vi "Example Code.vi"   [LabVIEW 2016]
uses:
  <vilib>/Skyline/Configuration/Configuration HTTP_class/Open Configuration HTTP.vi
  <vilib>/Skyline/Message/HTTP Wrapper/Open (HTTP).vi
  <vilib>/Skyline/Message/HTTP Wrapper/NI Skyline Message HTTP.lvclass
  <vilib>/Skyline/Configuration/Configuration HTTP_class/NI Skyline Configuration HTTP.lvclass
  <vilib>/Skyline/Message/NI Skyline Message.lvclass
  <vilib>/Skyline/Configuration/Configuration_class/NI Skyline Configuration.lvclass
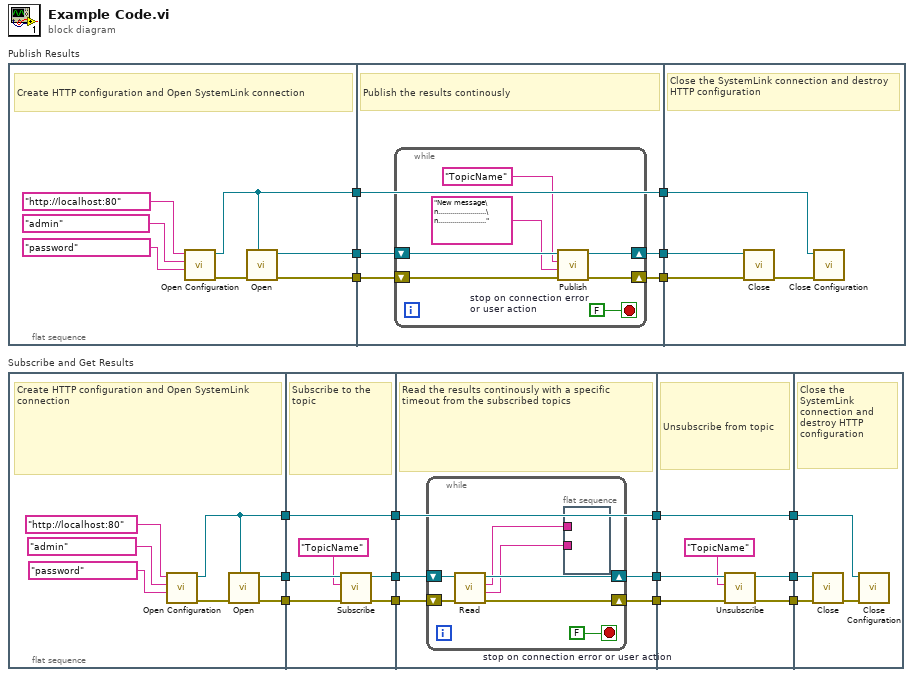
[diagram p0: block diagram]
diagram:
  n1 = flat-sequence "Publish Results" {
    tunnel: [w21] -> w18
    tunnel: [w20] -> w17
    tunnel: [w19] -> w16
    tunnel: w18 -> [w30]
    tunnel: w17 -> [w29]
    tunnel: w16 -> [w28]
    tunnel: [w28] -> w15
    tunnel: [w27] -> w14
    tunnel: [w26] -> w13
    tunnel: w15 -> [w38]
    tunnel: w14 -> [w39]
    tunnel: w13 -> [w40]
    frame #0 {
      # "Create HTTP configuration and Open SystemLink connection"
      n2 = call-poly <vilib>:"Open Configuration.vi"("password"="password", "username"="admin", "server url"="http://localhost:80") -> ("error out"=w25:errorcluster, "HTTP configuration out"=w19:refnum<class "NI Skyline Configuration HTTP.lvclass">)  [unwired: 7 in]
      n3 = call-poly <vilib>:"Open.vi"("configuration"=w19, "error in (no error)"=w25) -> ("error out"=w20:errorcluster, "message http out"=w21:refnum<class "NI Skyline Message HTTP.lvclass">)  [unwired: 8 in]
    }
    frame #1 {
      # "Publish the results continously"
      n4 = while {
        shift-right: [w35] -> w26
        shift-left: w30 -> [w37]
        shift-right: [w34] -> w27
        shift-left: w29 -> [w36]
        stop <- w31 stop-if-true
        w31 = FALSE  # stop on connection error or user action
        n5 = call-dynamic "Publish.vi"("error in (no error)"=w36, "message"="New message\n........................\n........................" ("topic"), "topic"="TopicName", "message http"=w37) -> ("error out"=w34:errorcluster, "message http out"=w35:refnum<class "NI Skyline Message HTTP.lvclass">)  [unwired: 6 in]
      }
    }
    frame #2 {
      # "Close the SystemLink connection and destroy HTTP configuration"
      n6 = call-dynamic "Close.vi"("error in (no error)"=w39, "message http"=w40) -> ("error out"=w41:errorcluster)  [unwired: 9 in]
      n7 = call-dynamic "Close Configuration.vi"("error in (no error)"=w41, "HTTP configuration in"=w38) -> ()  [unwired: 9 in, 1 out]
    }
  }
  n8 = flat-sequence "Subscribe and Get Results" {
    tunnel: [w44] -> w6
    tunnel: [w43] -> w5
    tunnel: [w42] -> w3
    tunnel: w6 -> [w53]
    tunnel: w5 -> [w52]
    tunnel: [w51] -> w4
    tunnel: w3 -> [w54]
    tunnel: [w54] -> w2
    tunnel: [w50] -> w1
    tunnel: w4 -> [w58]
    tunnel: w2 -> [w57]
    tunnel: [w57] -> w12
    tunnel: [w56] -> w10
    tunnel: [w55] -> w8
    tunnel: w1 -> [w59]
    tunnel: w12 -> [w72]
    tunnel: [w72] -> w11
    tunnel: w10 -> [w69]
    tunnel: [w68] -> w9
    tunnel: w8 -> [w71]
    tunnel: [w70] -> w7
    tunnel: w11 -> [w73]
    tunnel: w9 -> [w74]
    tunnel: w7 -> [w75]
    frame #0 {
      # "Create HTTP configuration and Open SystemLink connection"
      n9 = call-poly <vilib>:"Open Configuration.vi"("password"="password", "username"="admin", "server url"="http://localhost:80") -> ("error out"=w48:errorcluster, "HTTP configuration out"=w42:refnum<class "NI Skyline Configuration HTTP.lvclass">)  [unwired: 7 in]
      n10 = call-poly <vilib>:"Open.vi"("configuration"=w42, "error in (no error)"=w48) -> ("error out"=w43:errorcluster, "message http out"=w44:refnum<class "NI Skyline Message HTTP.lvclass">)  [unwired: 8 in]
    }
    frame #1 {
      # "Subscribe to the topic"
      n11 = call-dynamic "Subscribe.vi"("error in (no error)"=w52, "topic"="TopicName", "message http"=w53) -> ("error out"=w51:errorcluster, "message http out"=w50:refnum<class "NI Skyline Message HTTP.lvclass">)  [unwired: 7 in]
    }
    frame #2 {
      # "Read the results continously with a specific timeout from the subscribed topics"
      n12 = while {
        shift-right: [w64] -> w55
        shift-left: w59 -> [w66]
        shift-right: [w63] -> w56
        shift-left: w58 -> [w65]
        stop <- w62 stop-if-true
        w62 = FALSE  # stop on connection error or user action
        n13 = call-dynamic "Read.vi"("error in (no error)"=w65, "message http"=w66) -> ("error out"=w63:errorcluster, "message"=w60:string, "topic"=w61:string, "message http out"=w64:refnum<class "NI Skyline Message HTTP.lvclass">)  [unwired: 5 in, 1 out]
        n14 = flat-sequence {
          tunnel: w61 -> [_]
          tunnel: w60 -> [_]
          frame #0 {
          }
        }
      }
    }
    frame #3 {
      # "Unsubscribe from topic"
      n15 = call-dynamic "Unsubscribe.vi"("error in (no error)"=w69, "topic"="TopicName", "message http"=w71) -> ("error out"=w68:errorcluster, "message http out"=w70:refnum<class "NI Skyline Message HTTP.lvclass">)  [unwired: 7 in]
    }
    frame #4 {
      # "Close the SystemLink connection and destroy HTTP configuration"
      n16 = call-dynamic "Close.vi"("error in (no error)"=w74, "message http"=w75) -> ("error out"=w76:errorcluster)  [unwired: 9 in]
      n17 = call-dynamic "Close Configuration.vi"("error in (no error)"=w76, "HTTP configuration in"=w73) -> ()  [unwired: 9 in, 1 out]
    }
  }
